vi "Process Stopped Event.vi"() -> (3 "Process Stopped":refnum<user-event>)   [LabVIEW 2020]
uses:
  Process Stopped Cluster.ctl
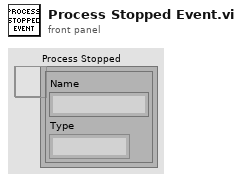
[diagram p1: front panel]
types:
  T1 = typedef "Process Stopped Cluster.ctl" = cluster{"Name":string, "Type":enum16{"Hardware", "Optimizer", "Analyzer"}}
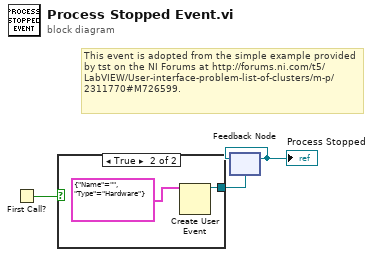
[diagram p0: block diagram]
diagram:
  # "This event is adopted from the simple example provided by tst on the NI Forums at http://forums.ni.com/t5/LabVIEW/User-interface-problem-list-of-clusters/m-p/2311770#M726599."
  n1 = First Call?() -> (First Call?: T/F=w3:bool)
  n2 = case shown="True" w3 {
    tunnel: [_ w5] -> w2
    frame False {
    }
    frame True {
      n3 = Create User Event(user event datatype=T1 {"Name"="", "Type"=enum."Hardware"} ("Process Cluster")) -> (user event=w5:refnum<user-event>)  [unwired: 1 in, 1 out]
    }
  }
  n4 = feedback #1(w2) -> (w1:refnum<user-event>)
  "Process Stopped" <- w1
  n5 = feedback-in #1(w1) -> ()
